vi "Check Close File.vi"(8 "error in (no error)":errorcluster, 11 "Segmented Log in":refnum<class "Segmented Log.lvclass">) -> (0 "error out":errorcluster, 3 "Segmented Log out":refnum<class "Segmented Log.lvclass">)   [LabVIEW 2012, in "Waveform Data Logger Engine.lvlib" / "Segmented Log.lvclass"]
doc: "Determine if the current log file instance needs to be closed and close it if so."
uses:
  Segmented Log.lvclass
  Segmented Log.lvclass/Segmented Log.ctl
  On Segmented Log Complete.vi
  On File Close.vi
  Log Files/Log File/Close Log File.vi
  Make File Read-Only.vi
  Log Files/Log File/Log File.lvclass
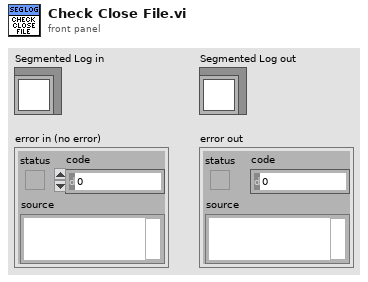
[diagram p1: front panel]
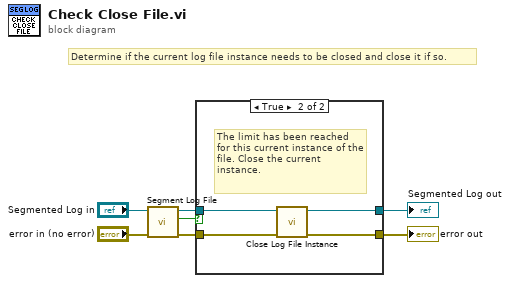
[diagram p0: block diagram]
diagram:
  # "Determine if the current log file instance needs to be closed and close it if so."
  n1 = call "Segment Log File.vi"("error in (no error)"="error in (no error)", "Segmented Log in"="Segmented Log in") -> ("error out"=w6:errorcluster, "Segment Log File"=w5:bool, "Segmented Log out"=w7:refnum<class "Segmented Log.lvclass">)  [unwired: 7 in]
  n2 = case shown="True" w5 {
    tunnel: w6 -> [w8 w13]
    tunnel: w7 -> [w9 w12]
    tunnel: [w9 w11] -> w2
    tunnel: [w8 w10] -> w1
    frame False {
    }
    frame True {
      # "The limit has been reached for this current instance of the file. Close the current instance."
      n3 = call "Close Log File Instance.vi"("error in (no error)"=w13, "Segmented Log in"=w12) -> ("error out"=w10:errorcluster, "Segmented Log out"=w11:refnum<class "Segmented Log.lvclass">)  [unwired: 8 in]
    }
  }
  "Segmented Log out" <- w2
  "error out" <- w1
